vi "Main.vi"() -> ()   [LabVIEW 2017, in "WebServiceImporter.lvlib" / "Main Panel.lvlib" / "Select Methods.lvlib"]
uses:
  <vilib>/Platform/WebService/Main Panel/Pages/Select Methods/Select Methods.lvlib
  <vilib>/Platform/WebService/Main Panel/Pages/Select Methods/Events/Events.lvlib
  <vilib>/Platform/WebService/VI Generator/VI Generator.lvlib
  <vilib>/Platform/WebService/Main Panel/Events/Events.lvlib
panel:
  in  "Panel":enum32{"Interface Frame", "Hidden Controls"}(tab)
  in  "UnCheck":bool
  in  "Check":bool
  in  "UnCheck All":bool
  in  "Check All":bool
  in  "Select Methods to Import":i32[](listbox)
  # "Select the methods to import"
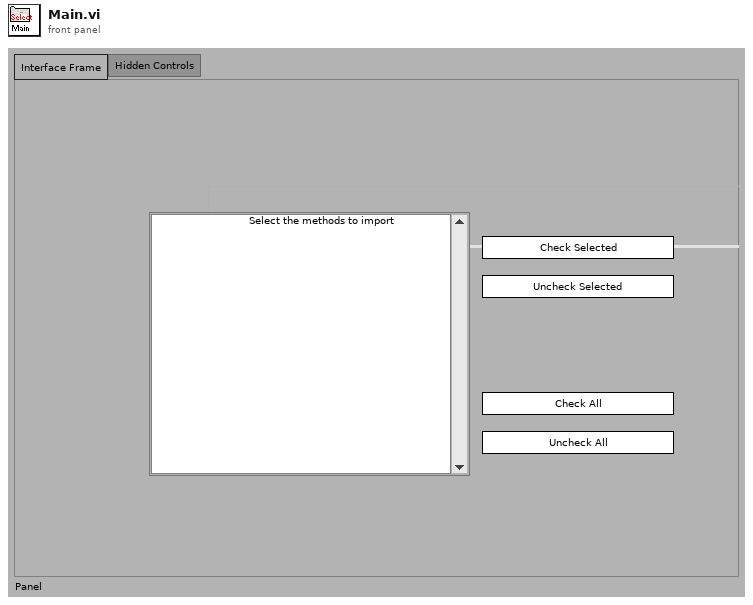
[diagram p1: front panel]
types:
  T1 = typedef "LVPoint32TypeDef.ctl" = cluster{"Horizontal":i32, "Vertical":i32}
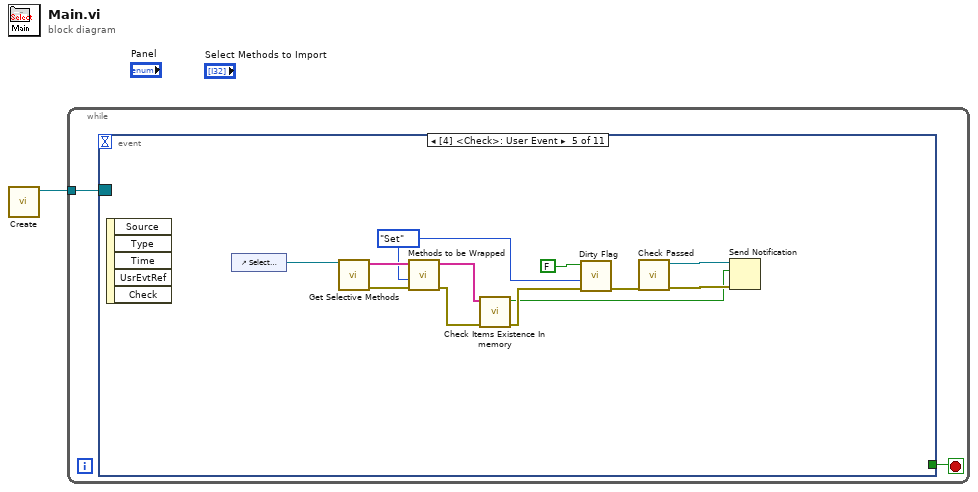
[diagram p0: block diagram]
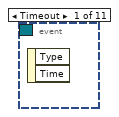
[diagram p2: hidden frame]
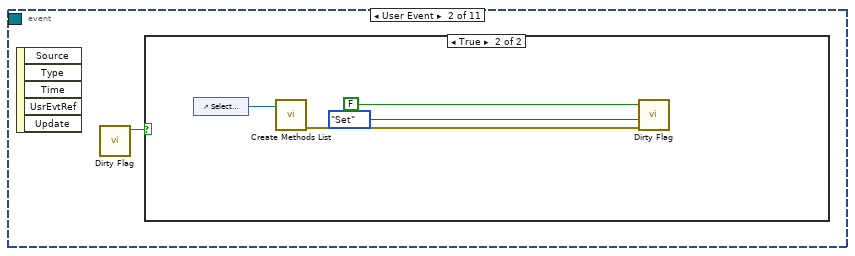
[diagram p3: hidden frame]
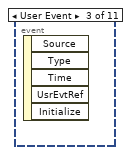
[diagram p5: hidden frame]
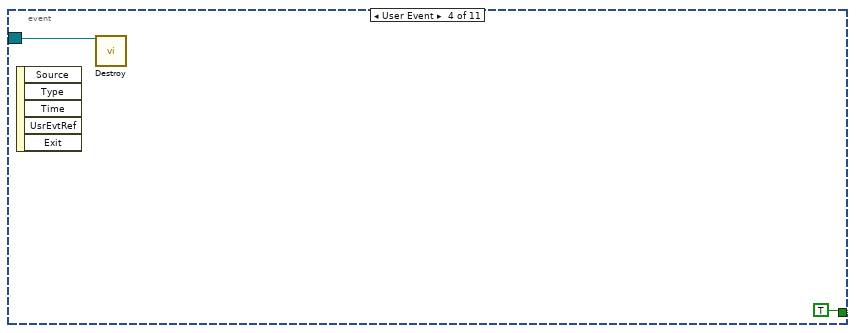
[diagram p6: hidden frame]
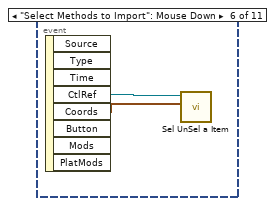
[diagram p7: hidden frame]
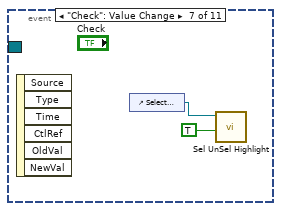
[diagram p8: hidden frame]
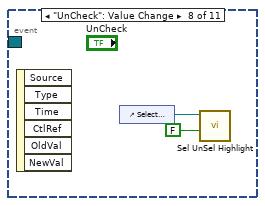
[diagram p9: hidden frame]
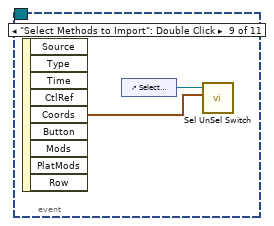
[diagram p10: hidden frame]
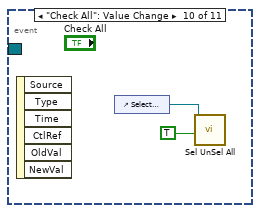
[diagram p11: hidden frame]
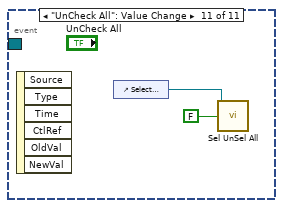
[diagram p12: hidden frame]
diagram:
  n1 = call <vilib>:"Create.vi"() -> ("Event Registration Refnum"=w1:refnum<event-registration>)  [unwired: 1 in, 10 out]
  n2 = while {
    tunnel: w1 -> [w3]
    stop <- w2 stop-if-true
    n3 = event shown="[4] <Check>: User Event" {
      selector: w3 -> [_ _ _ w10 _ _ _ _ _ _ _]
      dyn-events: _ -> [_ _ _ _ _ _ _ _ _ _ _]
      timeout: _ -> [_ _ _ _ _ _ _ _ _ _ _]
      tunnel: [_ _ _ TRUE _ _ _ _ _ _ _] -> w2
      event Timeout {
        n4 = event-data() -> ()  [unwired: 3 out]
      }
      event User Event {
        n5 = event-data() -> ()  [unwired: 6 out]
        n6 = call <vilib>:"Dirty Flag.vi"() -> ("Dirty (out)"=w4:bool)  [unwired: 3 in, 8 out]
        n7 = case shown="True" w4 {
          frame False {
          }
          frame True {
            n8 = control-ref of="Select Methods to Import"() -> (w5:refnum<vi>)
            n9 = call <vilib>:"Create Methods List.vi"("Methods ListCtrl"=w5) -> ("error out"=w6:errorcluster)  [unwired: 1 in, 9 out]
            n10 = call <vilib>:"Dirty Flag.vi"("error in (no error)"=w6, "Operation"=enum16{"Get", "Set"}."Set", "Dirty"=FALSE) -> ()  [unwired: 9 out]
          }
        }
      }
      event User Event {
        n11 = event-data() -> ()  [unwired: 6 out]
      }
      event User Event {
        n12 = event-data() -> ()  [unwired: 6 out]
        n13 = call <vilib>:"Destroy.vi"("Event Registration Refnum"=w10) -> ()  [unwired: 1 in, 10 out]
      }
      event User Event {
        w19 = enum16{"Get", "Set"}."Set" ("Operation")
        n14 = event-data() -> ()  [unwired: 6 out]
        n15 = control-ref of="Select Methods to Import"() -> (w21:refnum<vi>)
        n16 = call <vilib>:"Get Selective Methods.vi"("Methods ListCtrl"=w21) -> ("error out"=w17:errorcluster, "Selective Methods"=w22:string[])  [unwired: 1 in, 8 out]
        n17 = call <vilib>:"Methods to be Wrapped.vi"("error in (no error)"=w17, "Operation"=w19, "Methods to be Wrapped"=w22) -> ("error out"=w14:errorcluster, "Methods to be Wrapped (out)"=w12:string[])  [unwired: 7 out]
        n18 = call <vilib>:"Check Items Existence In memory.vi"("error in (no error)"=w14, "Methods to be Wrapped"=w12) -> ("error out"=w13:errorcluster, "Notify?"=w11:bool)  [unwired: 8 out]
        n19 = call <vilib>:"Dirty Flag.vi"("error in (no error)"=w13, "Operation"=w19, "Dirty"=FALSE) -> ("error out"=w16:errorcluster)  [unwired: 8 out]
        n20 = call <vilib>:"Check Passed.vi"("error in (no error)"=w16) -> ("error out"=w15:errorcluster, "notifier  (out)"=w20:refnum<notifier>)  [unwired: 2 in, 7 out]
        n21 = Send Notification(notification=w11, notifier=w20, error in (no error)=w15) -> ()  [unwired: 2 out]
      }
      event "Select Methods to Import": Mouse Down {
        n22 = event-data() -> ("CtlRef"=w24:refnum<vi>, "Coords"=w23:T1)  [unwired: 7 out]
        n23 = call <vilib>:"Sel UnSel a Item.vi"("Coords"=w23, "Methods ListCtrl"=w24) -> ()  [unwired: 1 in, 9 out]
      }
      event "Check": Value Change {
        n24 = event-data() -> ()  [unwired: 7 out]
        n25 = control-ref of="Select Methods to Import"() -> (w26:refnum<vi>)
        n26 = call <vilib>:"Sel UnSel Highlight.vi"("Check All? (T)"=TRUE, "Methods ListCtrl"=w26) -> ()  [unwired: 1 in, 9 out]
      }
      event "UnCheck": Value Change {
        n27 = event-data() -> ()  [unwired: 7 out]
        n28 = control-ref of="Select Methods to Import"() -> (w28:refnum<vi>)
        n29 = call <vilib>:"Sel UnSel Highlight.vi"("Check All? (T)"=FALSE, "Methods ListCtrl"=w28) -> ()  [unwired: 1 in, 9 out]
      }
      event "Select Methods to Import": Double Click {
        n30 = event-data() -> ("Coords"=w29:T1)  [unwired: 9 out]
        n31 = control-ref of="Select Methods to Import"() -> (w30:refnum<vi>)
        n32 = call <vilib>:"Sel UnSel Switch.vi"("Point"=w29, "Methods ListCtrl"=w30) -> ()  [unwired: 1 in, 9 out]
      }
      event "Check All": Value Change {
        n33 = event-data() -> ()  [unwired: 7 out]
        n34 = control-ref of="Select Methods to Import"() -> (w31:refnum<vi>)
        n35 = call <vilib>:"Sel UnSel All.vi"("Check All? (T)"=TRUE, "Methods ListCtrl"=w31) -> ()  [unwired: 1 in, 9 out]
      }
      event "UnCheck All": Value Change {
        n36 = event-data() -> ()  [unwired: 7 out]
        n37 = control-ref of="Select Methods to Import"() -> (w34:refnum<vi>)
        n38 = call <vilib>:"Sel UnSel All.vi"("Check All? (T)"=FALSE, "Methods ListCtrl"=w34) -> ()  [unwired: 1 in, 9 out]
      }
    }
  }
